vi "Reset.vi"(8 "error in (no error)":errorcluster, 10 "firmware revision":string, 11 "VISA resource name":refnum<visa-resource-name>) -> (0 "error out":errorcluster, 3 "VISA resource name out":refnum<visa-resource-name>)   [LabVIEW 2019, in "Andeen-Hagerling 2700A.lvlib"]
doc: "Resets the instrument and delay to allow the bridge time to reset."
uses:
  Andeen-Hagerling 2700A.lvlib
  Instance           1 13Saved   Reset .vi
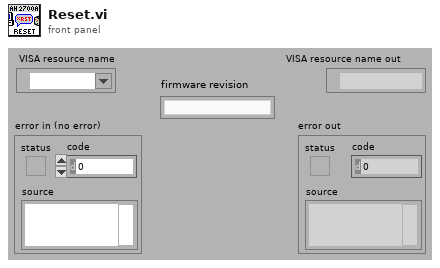
[diagram p1: front panel]
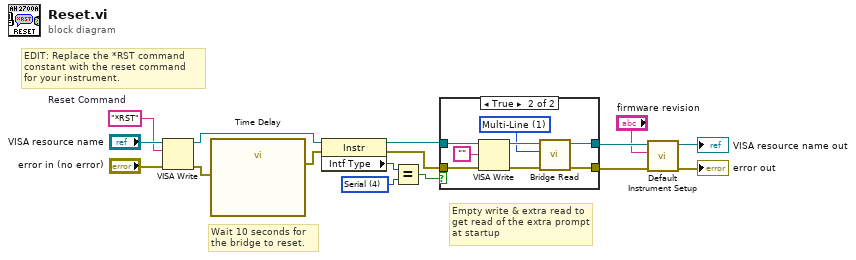
[diagram p0: block diagram]
diagram:
  w12 = u16 4 items=["GPIB"=1, "VXI"=2, "GPIB-VXI"=3, "Serial"=4, "PXI"=5, "TCPIP"=6, "USB"=7] ("Interface Information:Interface Type")
  w14 = "*RST"  # Reset Command
  # "Empty write & extra read to\nget read of the extra prompt\nat startup"
  # "Wait 10 seconds for\nthe bridge to reset."
  # "EDIT: Replace the *RST command\nconstant with the reset command\nfor your instrument."
  n1 = VISA Write(VISA resource name="VISA resource name", write buffer=w14, error in (no error)="error in (no error)") -> (VISA resource name out=w9:refnum<visa-resource-name>, error out=w13:errorcluster)  [unwired: 1 out]
  n2 = call "Time Delay"("error in (no error)"=w13) -> ("error out"=w10:errorcluster)  [unwired: 10 in]
  n3 = property class="Instr"(reference=w9, error in=w10) -> (reference out=w6:refnum<visa-resource-name>, error out=w4:errorcluster, "Intf Type"=w11:u16)
  n4 = Equal?(x=w11, y=w12) -> (x = y?=w5:bool)
  n5 = case shown="True" w5 {
    tunnel: w6 -> [w18 w25]
    tunnel: w4 -> [w17 w24]
    tunnel: [w18 w23] -> w3
    tunnel: [w17 w22] -> w2
    frame False {
    }
    frame True {
      w19 = u16 1 items=["Single Line", "Multi-Line"] ("Multiline")
      n6 = VISA Write(VISA resource name=w25, write buffer="", error in (no error)=w24) -> (VISA resource name out=w21:refnum<visa-resource-name>, error out=w20:errorcluster)  [unwired: 1 out]
      n7 = call "Bridge Read.vi"("error in (no error)"=w20, "multiline"=w19, "VISA resource name"=w21) -> ("error out"=w22:errorcluster, "VISA resource name out"=w23:refnum<visa-resource-name>)  [unwired: 6 in, 1 out]
    }
  }
  n8 = call "Default Instrument Setup.vi"("error in (no error)"=w2, "firmware revision"="firmware revision", "VISA resource name"=w3) -> ("error out"=→"error out":errorcluster, "VISA resource name out"=→"VISA resource name out":refnum<visa-resource-name>)  [unwired: 7 in]
